vi "webPublishing.vi"() -> ()   [LabVIEW 2014]
panel:
  out "Numeric 2":dbl
  out "Numeric":dbl
  in  "stop":bool
  out "Boolean 2":bool
  in  "Boolean":bool
  in  "Slide 2":dbl(slide) scale=0.0..100.0
  out "Slide":dbl(slide) scale=0.0..100.0
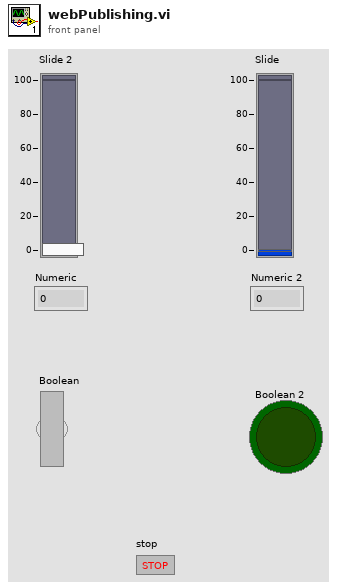
[diagram p1: front panel]
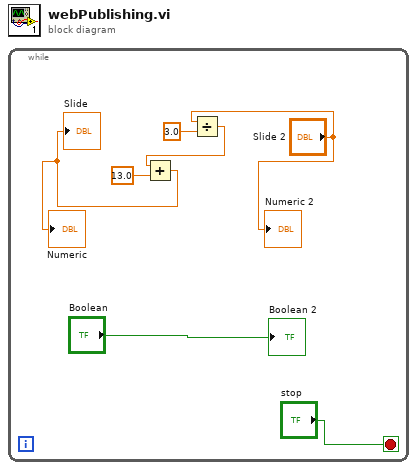
[diagram p0: block diagram]
diagram:
  n1 = while {
    stop <- "stop" stop-if-true
    n2 = Divide(x="Slide 2", y=3.0) -> (x/y=w3:dbl)
    n3 = Add(x=w3, y=13.0) -> (x+y=→"Slide" →"Numeric":dbl)
    "Boolean 2" <- "Boolean"
    "Numeric 2" <- "Slide 2"
  }
